vi "Write Register.vi"(8 "Error In":errorcluster, 9 "Data":u8, 10 "Register Address":u8, 11 "Adept Config":T1) -> (0 "Error Out":errorcluster, 3 "Adept Config":T1)   [LabVIEW 2011, in "LVH-Adept.lvlib"]
uses:
  <vilib>/LabVIEW Hacker/Adept/LVH-Adept.lvlib
  <vilib>/LabVIEW Hacker/Adept/Private/Type Defs/Device Config.ctl
  <vilib>/LabVIEW Hacker/Adept/Private/DPCUTIL/DPCUTIL.lvlib
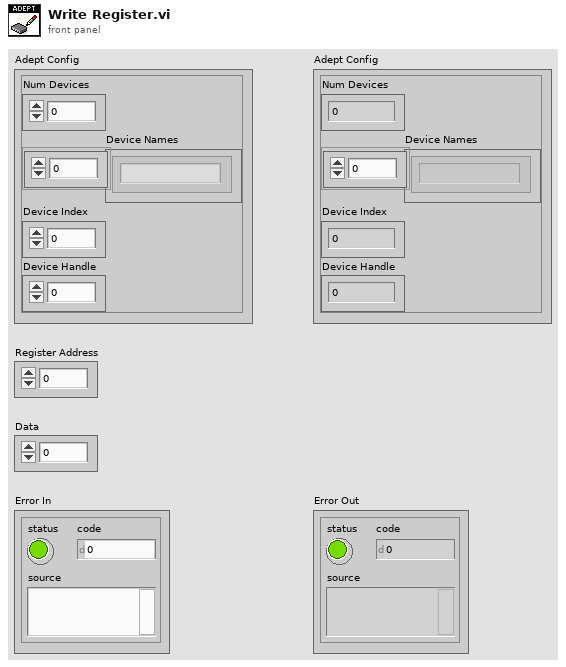
[diagram p1: front panel]
types:
  T1 = typedef "LVH-Adept.lvlib/Device Config.ctl" = cluster{"Num Devices":i32, "Device Names":string[], "Device Index":u16, "Device Handle":u32}
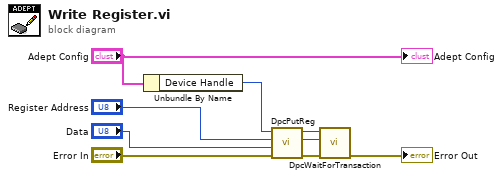
[diagram p0: block diagram]
diagram:
  n1 = Unbundle By Name("Adept Config") -> ("Device Handle"=w8:u32)
  n2 = call <vilib>:"DpcPutReg.vi"("Error In"="Error In", "Data"="Data", "Register Address"="Register Address", "Device Handle"=w8) -> ("Error Out"=w5:errorcluster, "Task ID"=w3:u16, "Device Hanle"=w4:u32)  [unwired: 5 in]
  n3 = call <vilib>:"DpcWaitForTransaction.vi"("Error In"=w5, "Task ID"=w3, "Device Handle"=w4) -> ("Error Out"=→"Error Out":errorcluster)  [unwired: 7 in, 1 out]
  "Adept Config" <- "Adept Config"
